vi "Assert Array Distinct.vi"(4 "Execution time (s)":dbl=-1.0, 5 "Assert Only? (F)":bool, 6 "error code (1)":i32=1, 7 "Label (\"\")":string, 8 "error in (no error)":errorcluster, 9 "Register with caller test (F)":bool, 11 "Array":variant) -> (0 "error out":errorcluster, 2 "Properties.Assert":refnum<class "Properties.Assert.lvclass">)   [LabVIEW 2013, in "Caraya.lvlib" / "Assert.lvclass"]
doc: "Asserts that an array contains each element only once."
uses:
  Assert.lvclass
  Properties.Assert/Properties.Assert.lvclass
  Properties/Properties.lvclass
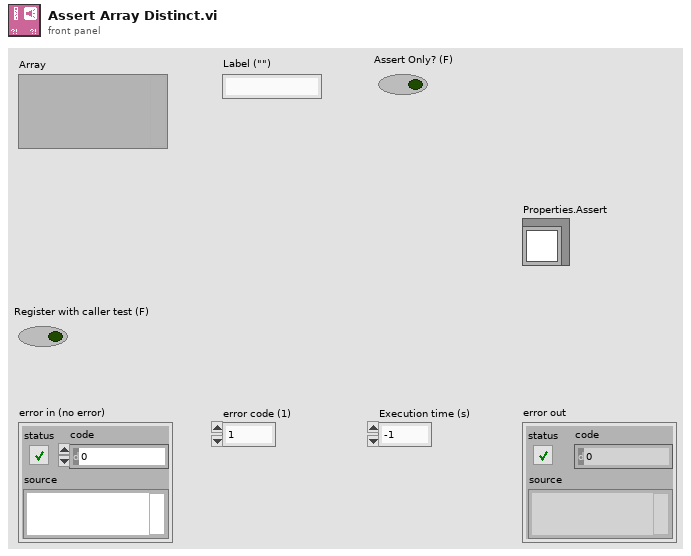
[diagram p1: front panel]
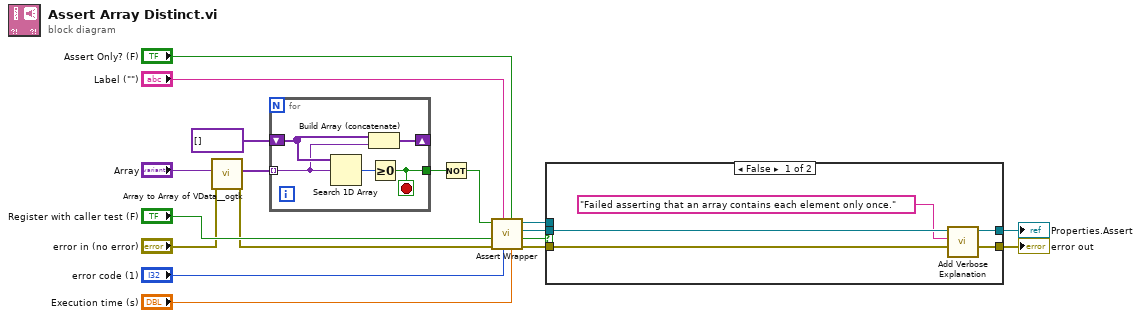
[diagram p0: block diagram]
diagram:
  n1 = call <userlib>:"Array to Array of VData__ogtk.vi"("error in (no error)"="error in (no error)", "MultiD Array"="Array") -> ("error out"=w5:errorcluster, "1D Array of Variants"=w4:variant[])  [unwired: 8 in]
  n2 = for {
    tunnel: w4 -> [w21] mode=indexing
    shift-right: [w23] -> _
    shift-left: variant[] [] -> [w22]
    tunnel: [w19] -> w3
    stop <- w19 stop-if-true
    n3 = Search 1D Array(1D array=w22, element=w21) -> (index of element=w20:i32)  [unwired: 1 in]
    n4 = Build Array (concatenate)(w22, w21) -> (w23:variant[])
    n5 = Greater Or Equal To 0?(x=w20) -> (x >= 0?=w19:bool)
  }
  n6 = Not(x=w3) -> (.not. x?=w2:bool)
  n7 = call "Assert Wrapper.vi"("Execution time (s)"="Execution time (s)", "Assert Only? (F)"="Assert Only? (F)", "error code (1)"="error code (1)", "Label"="Label (\"\")", "error in (no error)"=w5, "Register with caller test (F)"="Register with caller test (F)", "Assert?"=w2) -> ("error out"=w9:errorcluster, "Verbose"=w13:bool, "Properties.Assert"=w11:refnum<class "Properties.Assert.lvclass">, "Assert out"=w12:refnum<class "Assert.lvclass">)  [unwired: 1 in]
  n8 = case shown="False" w13 {
    tunnel: w12 -> [_ _]
    tunnel: w11 -> [w26 w30]
    tunnel: [w27 w29] -> w10
    tunnel: w9 -> [w28 w29]
    tunnel: [w25 w30] -> w8
    frame False {
      n9 = call "Add Verbose Explanation.vi"("error in (no error)"=w28, "Verbose Explanation"="Failed asserting that an array contains each element only once.", "Properties"=w26) -> ("error out"=w27:errorcluster, "Properties"=w25:refnum<class "Properties.Assert.lvclass">)  [unwired: 7 in]
    }
    frame True {
    }
  }
  "error out" <- w10
  "Properties.Assert" <- w8
